vi "Product_PCU.vi"() -> ()   [LabVIEW 2017]
panel:
  in  "Product_PCU":enum32{"rdopcu100", "rdopcu110"}(radio) caption="Product"
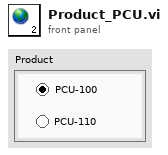
[diagram p1: front panel]
diagram:
